vi "GetMUXStatus.vi"(8 "error in (no error)":errorcluster, 10 "gRPCid":T2, 11 "ctet_mux in":T1) -> (0 "error out":errorcluster, 3 "ctet_mux out":T1)   [LabVIEW 2019, in "ctet_mux_User Library.lvlib"]
uses:
  ctet_mux_User Library.lvlib
  Servers/ctet_mux/gRPC lvSupport/Server API/typeDefs/grpcId.ctl
  Types/ctet_mux.ctl
  Servers/ctet_mux/ctet_mux Class/RPC Messages/measurementservice_MUXGetStatusResponse/measurementservice_MUXGetStatusResponse_Data.ctl
  Servers/ctet_mux/ctet_mux Class/RPC Messages/measurementservice_ErrorOut/measurementservice_ErrorOut_Data.ctl
  Types/Switch Action.ctl
  Servers/ctet_mux/ctet_mux Class/ctet_mux.lvclass
  Servers/ctet_mux/gRPC lvSupport/gprc-lvsupport.lvlib
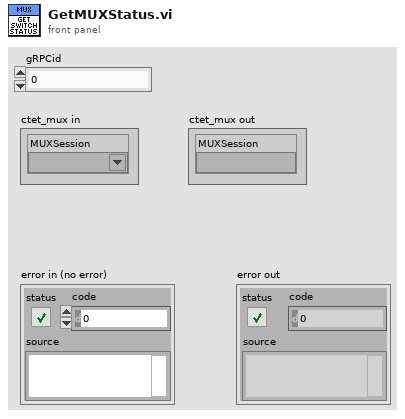
[diagram p1: front panel]
types:
  T1 = typedef "ctet_mux_User Library.lvlib/ctet_mux.ctl" = cluster{"MUXSession":refnum<k15>}
  T2 = typedef "ctet_mux.lvlib/gprc-lvsupport.lvlib/grpcId.ctl" = u64
  T3 = typedef "ctet_mux_User Library.lvlib/Switch Action.ctl" = enum16{"Get Switch State", "Initialize", "Connect Channel", "Open Channel", "Close Relay", "Open Relay", "Disconnect/Open All"}
  T4 = typedef "ctet_mux.lvlib/ctet_mux.lvclass/measurementservice_ErrorOut_Data.ctl" = cluster{"errCode":i64, "errMessage":string}
  T5 = typedef "ctet_mux.lvlib/ctet_mux.lvclass/measurementservice_MUXGetStatusResponse_Data.ctl" = cluster{"Status":string[], "error":T4}
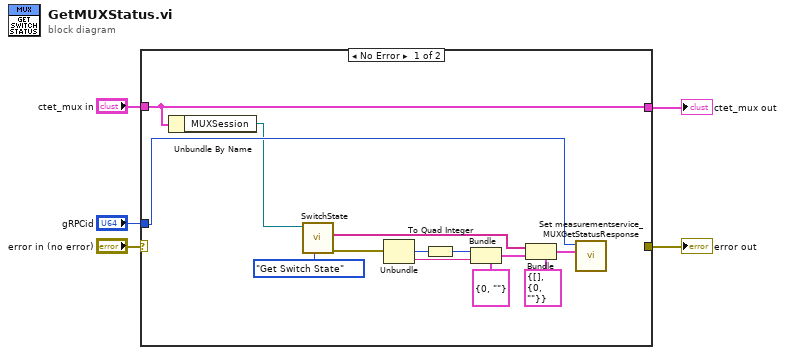
[diagram p0: block diagram]
diagram:
  n1 = case shown="No Error" "error in (no error)" {
    selector: "error in (no error)" -> [_ w20]
    tunnel: [_ w20] -> w5
    tunnel: "gRPCid" -> [w16 _]
    tunnel: "ctet_mux in" -> [w17 w19]
    tunnel: [w17 w19] -> w1
    frame No Error {
      n2 = Unbundle By Name(w17) -> ("MUXSession"=w11:refnum<k15>)
      n3 = call "SwitchState.vi"("Switch Action"=Switch_Action."Get Switch State", "Switch Session"=w11) -> ("error out"=w10:errorcluster, "Switch State"=w6:string[])  [unwired: 7 in, 1 out]
      n4 = Unbundle(w10) -> ("code"=w8:i32, "source"=w7:string)  [unwired: 1 out]
      n5 = To Quad Integer(1:w8) -> (0:w18:i64)
      n6 = Bundle(cluster=T4 {"errCode"=0, "errMessage"=""} ("error"), "errCode"=w18, "errMessage"=w7) -> (w12:T4)
      n7 = Bundle(cluster=T5 {"Status"=[], "error"={"errCode"=0, "errMessage"=""}} ("measurementservice_MUXGetStatusResponse_Data"), "Status"=w6, "error"=w12) -> (w14:T5)
      n8 = call "Set measurementservice_MUXGetStatusResponse.vi"("Message Data"=w14, "gRPCid"=w16) -> ()  [unwired: 9 in, 1 out]
    }
    frame Error {
    }
  }
  "error out" <- w5
  "ctet_mux out" <- w1
